vi "Close WF progress bar.vi"(8 "error in (no error)":errorcluster, 11 "ProgressBar_WireFlow in":refnum<class "ProgressBar_WireFlow.lvclass">) -> (0 "error out":errorcluster)   [LabVIEW 2013]
uses:
  <vilib>/addons/WireFlow/_WF_ProgressBar.llb/ProgressBar_WireFlow.lvclass
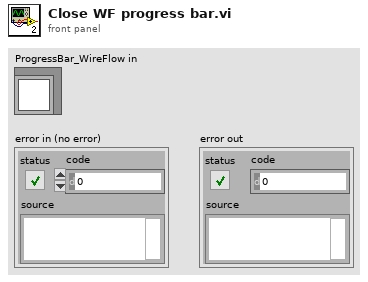
[diagram p1: front panel]
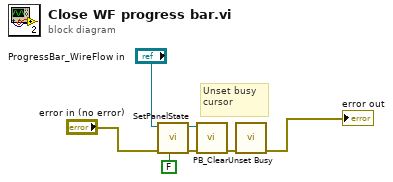
[diagram p0: block diagram]
diagram:
  # "Unset busy cursor"
  n1 = call-dynamic "SetPanelState.vi"("State (T = Open)"=FALSE, "error in (no error)"="error in (no error)", "WF-ProgressBar in"="ProgressBar_WireFlow in") -> ("error out"=w2:errorcluster, "WF-ProgressBar out"=w3:refnum<class "ProgressBar_WireFlow.lvclass">)  [unwired: 7 in]
  n2 = call-dynamic "PB_Clear.vi"("error in (no error)"=w2, "WF-ProgressBar in"=w3) -> ("error out"=w1:errorcluster)  [unwired: 8 in, 1 out]
  n3 = call <vilib>:"Unset Busy.vi"("error in (no error)"=w1) -> ("error out"=→"error out":errorcluster)  [unwired: 10 in]
